vi "Has Expired.vi"(1 "start time (ms)":u32, 2 "Timeout":T1={"mode"=enum."Relative", "deadline (ms)"=30000}) -> (0 "expired?":bool)   [LabVIEW 2020, in "NI_Deadline.lvlib"]
uses:
  <vilib>/Utility/Deadline/NI_Deadline.lvlib
  <vilib>/Utility/Deadline/Deadline.ctl
  <vilib>/Utility/Deadline/Mode.ctl
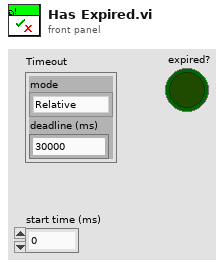
[diagram p1: front panel]
types:
  T1 = typedef "NI_Deadline.lvlib/Deadline.ctl" = cluster{"mode":T2, "deadline (ms)":u32}
  T2 = typedef "NI_Deadline.lvlib/Mode.ctl" = enum16{"Relative", "Use deadline", "Wait forever", "Nonblocking", "N/A"}
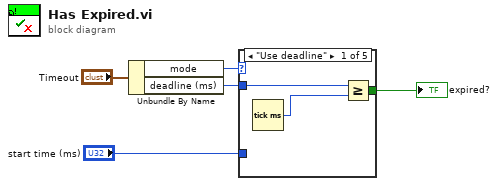
[diagram p0: block diagram]
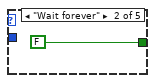
[diagram p2: hidden frame]
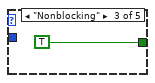
[diagram p3: hidden frame]
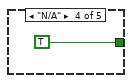
[diagram p4: hidden frame]
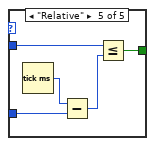
[diagram p5: hidden frame]
diagram:
  n1 = Unbundle By Name("Timeout") -> ("mode"=w4:T2, "deadline (ms)"=w3:u32)
  n2 = case shown="\"Use deadline\"" w4 {
    tunnel: w3 -> [w8 _ _ _ w14]
    tunnel: [w6 FALSE ("expired?") TRUE ("expired?") TRUE ("expired?") w12] -> w2
    tunnel: "start time (ms)" -> [_ _ _ _ w15]
    frame "Use deadline" {
      n3 = Tick Count (ms)() -> (millisecond timer value=w7:u32)
      n4 = Greater Or Equal?(x=w8, y=w7) -> (x >= y?=w6:bool)
    }
    frame "Wait forever" {
    }
    frame "Nonblocking" {
    }
    frame "N/A" {
    }
    frame "Relative" {
      n5 = Tick Count (ms)() -> (millisecond timer value=w16:u32)
      n6 = Subtract(x=w16, y=w15) -> (x-y=w13:u32)
      n7 = Less Or Equal?(x=w14, y=w13) -> (x <= y?=w12:bool)
    }
  }
  "expired?" <- w2
